vi "3P_Dischrg.vi"(0 "Parallel Task in":refnum<k21>, 1 "Capacity (Ah)":dbl format="%#.6g", 2 "C rate Setpoint":dbl format="%#.6g", 3 "Discharge Voltage Setpoint":dbl format="%#.6g", 5 "P task error in":errorcluster, 9 "NHR VISA in":refnum<visa-resource-name>, 11 "NHR error in":errorcluster caption="NHR error in (no error)", 12 "DischargeCyclePath":path=path "C:/Users/ga11/Desktop/VI/results/3PtestCharge.lvm" caption="Filename", 13 "Current Cutoff":dbl) -> (4 "parallel task out":refnum<k21>, 6 "parallel task error out":errorcluster, 10 "VISA resource name out":refnum<visa-resource-name>, 15 "NHR error out":errorcluster)   [LabVIEW 2020]
uses:
  <vilib>/DAQmx/read.llb/DAQmx Read (Analog 1D DBL NChan 1Samp).vi
  <vilib>/DAQmx/miscellaneous.llb/DAQmx Fill In Error Info.vi
  <instrlib>/NH Research Regenerative Test Series/Public/Data/Read (Ave Current).vi
  <instrlib>/NH Research Regenerative Test Series/Public/Data/Low Level/Fetch (Ave Voltage).vi
  <instrlib>/NH Research Regenerative Test Series/Public/Data/Low Level/Fetch (Ave True Power).vi
  <instrlib>/NH Research Regenerative Test Series/NH Research Regenerative Test Series.lvlib
panel:
  out "dischrge Ave Current (A)":dbl
  out "dischrg Ave Voltage (V)":dbl
  out "dischrg Ave True Power (W)":dbl
  out "Status Byte Register":T1
  out "Current Compare":dbl
  out "Battery1DischargeCurrent":dbl
  out "Battery2DischargeCurrent":dbl
  out "Battery3DischargeCurrent":dbl
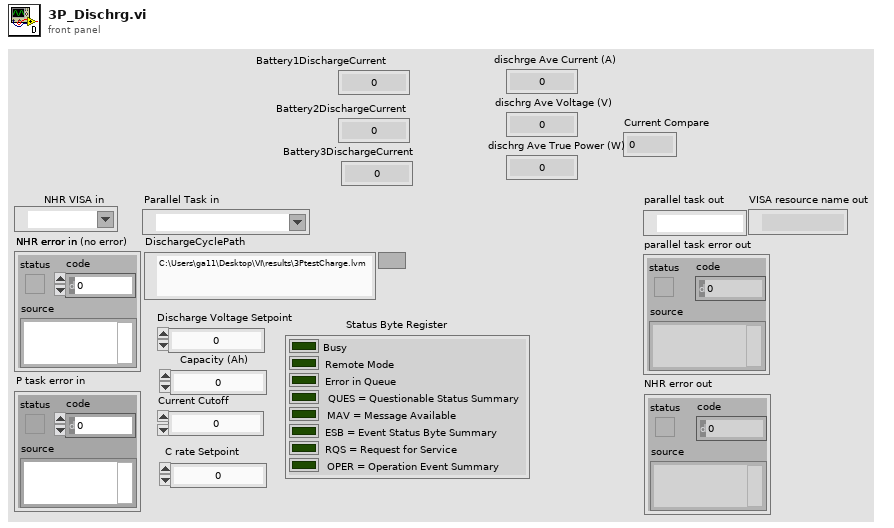
[diagram p1: front panel]
types:
  T1 = cluster{"Busy":bool, "Remote Mode":bool, "Error in Queue":bool, "QUES = Questionable Status Summary":bool, "MAV = Message Available":bool, "ESB = Event Status Byte Summary":bool, "RQS = Request for Service":bool, "OPER = Operation Event Summary":bool}
  T2 = cluster{"Voltage Enabled":bool, "Current Enabled":bool, "Power Enabled":bool, "Resistance Enabled":bool}
  T3 = cluster{"data[0]":dbl, "data[1]":dbl, "data[2]":dbl, "data[3]":dbl, "data[4]":dbl, "data[5]":dbl, "data[6]":dbl, "data[7]":dbl, "data[8]":dbl, "data[9]":dbl}
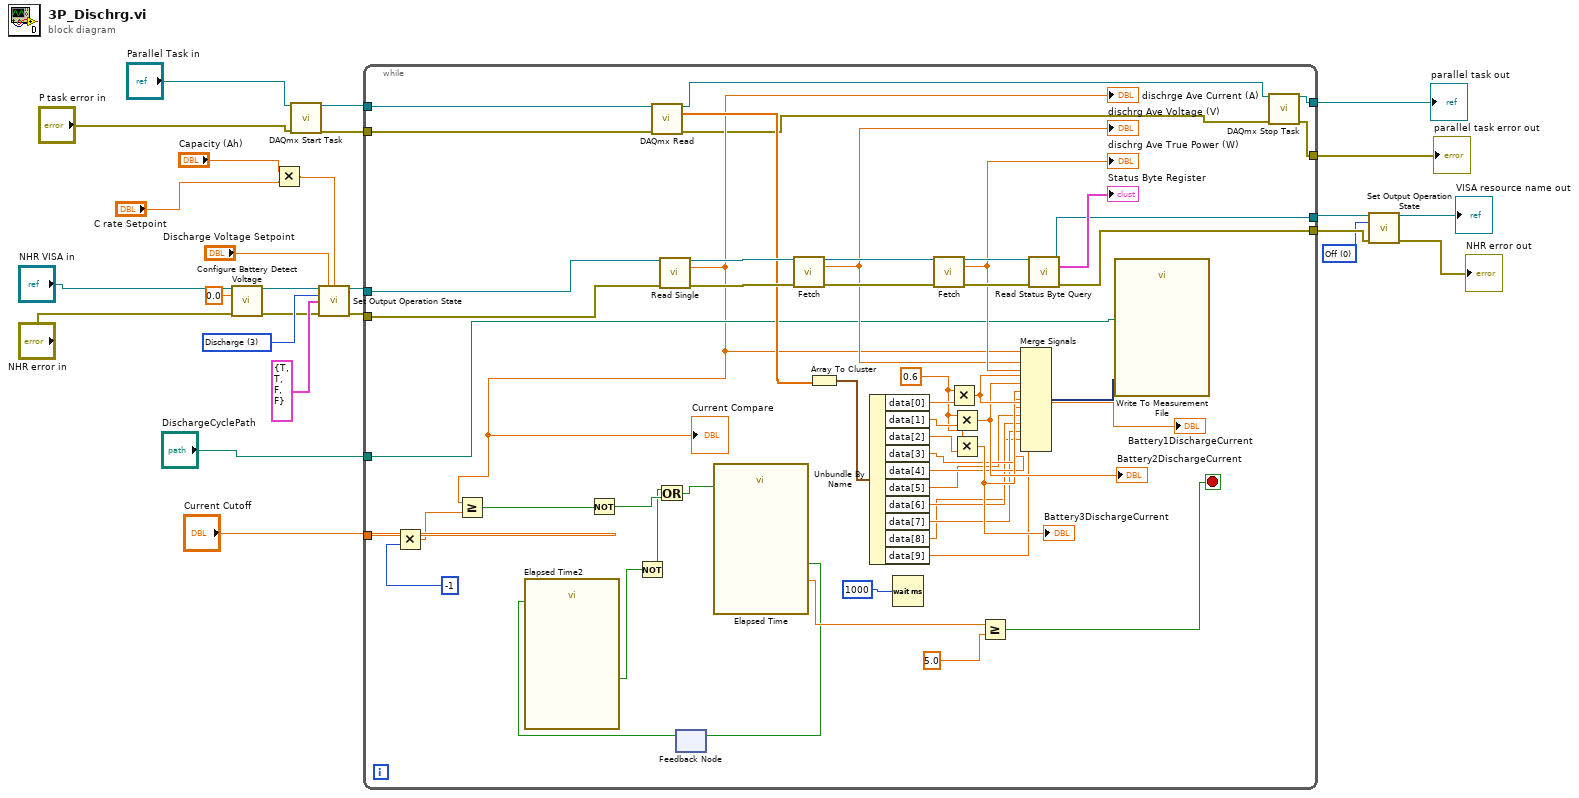
[diagram p0: block diagram]
diagram:
  w10 = 0 items=["Off", "Standby", "Charge", "Discharge", "Battery"] ("Mode (0: Off)")
  w18 = 3 items=["Off", "Standby", "Charge", "Discharge", "Battery"] ("Mode (0: Off)")
  n1 = call <instrlib>:"Configure Battery Detect Voltage.vi"("VISA resource name"="NHR VISA in", "Battery Detect Voltage (0V)"=0.0, "error in (no error)"="NHR error in") -> ("VISA resource name out"=w7:refnum<visa-resource-name>, "error out"=w6:errorcluster)  [unwired: 11 in]
  n2 = Multiply(x="Capacity (Ah)", y="C rate Setpoint") -> (x*y=w21:dbl)
  n3 = call <vilib>:"DAQmx Start Task.vi"("task/channels in"="Parallel Task in", "error in"="P task error in") -> ("task out"=w16:refnum<k21>, "error out"=w15:errorcluster)  [unwired: 12 in]
  n4 = call <vilib>:"Set Output Operation State.vi"("VISA resource name"=w7, "Voltage Setpoint (0 V)"="Discharge Voltage Setpoint", "Current Setpoint (0 A)"=w21, "Mode (0: Off)"=w18, "Enable"=T2 {"Voltage Enabled"=TRUE, "Current Enabled"=TRUE, "Power Enabled"=FALSE, "Resistance Enabled"=FALSE}, "error in (no error)"=w6) -> ("VISA resource name out"=w25:refnum<visa-resource-name>, "error out"=w24:errorcluster)  [unwired: 8 in]
  n5 = while {
    tunnel: w25 -> [w72]
    tunnel: w24 -> [w71]
    tunnel: [w69] -> w12
    tunnel: [w68] -> w11
    tunnel: "Current Cutoff" -> [w31]
    tunnel: w15 -> [w38]
    tunnel: w16 -> [w37]
    tunnel: "DischargeCyclePath" -> [w36]
    tunnel: [w28] -> w2
    tunnel: [w27] -> w1
    stop <- w41 stop-if-true
    w55 = 0.6
    n6 = Multiply(x=w31, y=-1) -> (x*y=w34:dbl)
    n7 = call-poly <vilib>:"DAQmx Read.vi"("task/channels in"=w37, "error in"=w38) -> ("task out"=w30:refnum<k21>, "data"=w66:dbl[], "error out"=w29:errorcluster)  [unwired: 11 in]
    n8 = call-poly <instrlib>:"Read Single.vi"("VISA resource name"=w72, "error in (no error)"=w71) -> ("VISA resource name out"=w77:refnum<visa-resource-name>, "Ave Current (A)"=w33:dbl, "error out"=w78:errorcluster)  [unwired: 11 in]
    "dischrge Ave Current (A)" <- w33
    "Current Compare" <- w33
    n9 = Greater Or Equal?(x=w33, y=w34) -> (x >= y?=w32:bool)
    n10 = Not(x=w32) -> (.not. x?=w47:bool)
    n11 = feedback #1() -> (w39:bool)  [unwired: 1 in]
    n12 = call "Elapsed Time2"("Reset"=w39) -> ("Time has Elapsed"=w46:bool)  [unwired: 11 in, 7 out]
    n13 = Not(x=w46) -> (.not. x?=w45:bool)
    n14 = Or(x=w45, y=w47) -> (x .or. y?=w44:bool)
    n15 = call "Elapsed Time"("Reset"=w44) -> ("Elapsed Time (s)"=w43:dbl, "Time has Elapsed"=w40:bool)  [unwired: 11 in, 6 out]
    n16 = feedback-in #1(w40) -> ()
    n17 = call-poly <instrlib>:"Fetch.vi"("VISA resource name"=w77, "error in (no error)"=w78) -> ("VISA resource name out"=w76:refnum<visa-resource-name>, "Ave Voltage (V)"=w63:dbl, "error out"=w75:errorcluster)  [unwired: 11 in]
    "dischrg Ave Voltage (V)" <- w63
    n18 = Array To Cluster(array=w66) -> (cluster=w65:T3)
    n19 = Unbundle By Name(w65) -> ("data[0]"=w61:dbl, "data[1]"=w59:dbl, "data[2]"=w56:dbl, "data[3]"=w54:dbl, "data[4]"=w53:dbl, "data[5]"=w52:dbl, "data[6]"=w51:dbl, "data[7]"=w50:dbl, "data[8]"=w49:dbl, "data[9]"=w48:dbl)
    n20 = Wait (ms)(milliseconds to wait=1000) -> ()  [unwired: 1 out]
    n21 = call-poly <instrlib>:"Fetch.vi"("VISA resource name"=w76, "error in (no error)"=w75) -> ("VISA resource name out"=w74:refnum<visa-resource-name>, "Ave True Power (W)"=w67:dbl, "error out"=w73:errorcluster)  [unwired: 11 in]
    "dischrg Ave True Power (W)" <- w67
    n22 = Multiply(x=w55, y=w61) -> (x*y=w60:dbl)
    "Battery1DischargeCurrent" <- w60
    n23 = Multiply(x=w55, y=w59) -> (x*y=w58:dbl)
    "Battery2DischargeCurrent" <- w58
    n24 = Multiply(x=w55, y=w56) -> (x*y=w57:dbl)
    "Battery3DischargeCurrent" <- w57
    n25 = Greater Or Equal?(x=w43, y=5.0) -> (x >= y?=w41:bool)
    n26 = Merge Signals "Merge Signals"(w33, w63, w67, w60, w58, w57, w54, w53, w52, w51, w50, w49, w48) -> (w64:dynamicdata)
    n27 = call <instrlib>:"Read Status Byte Query.vi"("VISA resource name"=w74, "error in (no error)"=w73) -> ("VISA resource name out"=w69:refnum<visa-resource-name>, "Status Byte Register"=→"Status Byte Register":T1, "error out"=w68:errorcluster)  [unwired: 11 in]
    n28 = call "Write To Measurement File"("Signals"=w64, "Filename"=w36) -> ()  [unwired: 15 in, 3 out]
    n29 = call <vilib>:"DAQmx Stop Task.vi"("task/channels in"=w30, "error in"=w29) -> ("task out"=w28:refnum<k21>, "error out"=w27:errorcluster)  [unwired: 12 in]
  }
  "parallel task out" <- w2
  "parallel task error out" <- w1
  n30 = call <vilib>:"Set Output Operation State.vi"("VISA resource name"=w12, "Mode (0: Off)"=w10, "error in (no error)"=w11) -> ("VISA resource name out"=→"VISA resource name out":refnum<visa-resource-name>, "error out"=→"NHR error out":errorcluster)  [unwired: 11 in]
